vi "Get SLSC Chassis ID.vi"(8 "error in (no error)":errorcluster, 11 "SLSC Chassis Ref in":T2 format="%.0x") -> (0 "error out":errorcluster, 2 "SLSC Chassis ID":T1 {"chassisType" items=["e12001_CHASSIS_TYPE"]; "ChassisIDType" items=["ChassisName", "HostnameIPAddress"]}, 3 "SLSC Chassis Ref out":T2 format="%.0x")   [LabVIEW 2020, in "VeriStand SLSC Scripting.lvlib"]
uses:
  VeriStand SLSC Scripting.lvlib
  <vilib>/NI VeriStand/Custom Device API/Custom Device Item Ref.ctl
  Controls/SLSC Chassis ID.ctl
  NationalInstruments.VeriStand.SystemDefinitionAPI
  <vilib>/NI VeriStand/Custom Device API/Custom Device API.lvlib
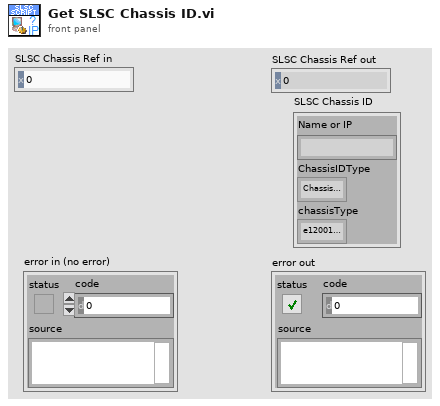
[diagram p1: front panel]
types:
  T1 = typedef "VeriStand SLSC Scripting.lvlib/SLSC Chassis ID.ctl" = cluster{"Name or IP":string, "ChassisIDType":i32, "chassisType":i32}
  T2 = typedef "Custom Device API.lvlib/Custom Device Item Ref.ctl" = u64
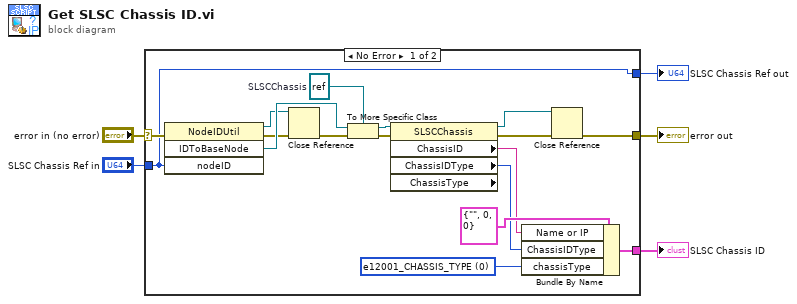
[diagram p0: block diagram]
diagram:
  n1 = case shown="No Error" "error in (no error)" {
    selector: "error in (no error)" -> [w13 w24]
    tunnel: [w17 w24] -> w5
    tunnel: "SLSC Chassis Ref in" -> [w12 w23]
    tunnel: [w12 w23] -> w2
    tunnel: [w10 _] -> w1
    frame No Error {
      w6 = 0 items=["e12001_CHASSIS_TYPE"] ("chassisType")
      w22 = refnum<k24> refnum  # SLSCChassis
      n2 = invoke class="NodeIDUtil" method="IDToBaseNode"(error in=w13, "nodeID"=w12) -> (reference out=w18:refnum<k24>, error out=w19:errorcluster, "IDToBaseNode"=w21:refnum<k24>)  [unwired: 2 in, 1 out]
      n3 = Close Reference(reference=w18, error in (no error)=w19) -> (error out=w20:errorcluster)
      n4 = To More Specific Class(target class=w22, reference=w21, error in=w20) -> (specific class reference=w8:refnum<k24>, error out=w16:errorcluster)
      n5 = property class="SLSCChassis" props=["ChassisID", "ChassisIDType", "ChassisType"](reference=w8, error in=w16) -> (reference out=w15:refnum<k24>, error out=w14:errorcluster, "ChassisID"=w9:string, "ChassisIDType"=w7:i32)  [unwired: 1 out]
      n6 = Bundle By Name(cluster=T1 {"Name or IP"="", "ChassisIDType"=0, "chassisType"=0} ("SLSC Chassis ID"), "Name or IP"=w9, "ChassisIDType"=w7, "chassisType"=w6) -> (w10:T1)
      n7 = Close Reference(reference=w15, error in (no error)=w14) -> (error out=w17:errorcluster)
    }
    frame Error {
    }
  }
  "error out" <- w5
  "SLSC Chassis Ref out" <- w2
  "SLSC Chassis ID" <- w1
